vi "UI_playerWins.vi"(8 "error in (no error)":errorcluster, 11 "Array":refnum<vi>[](array[refnum])) -> (0 "error out":errorcluster, 3 "win string":string)   [LabVIEW 2020]
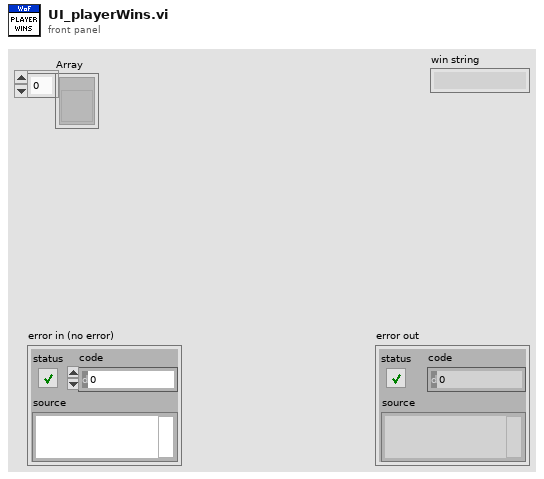
[diagram p1: front panel]
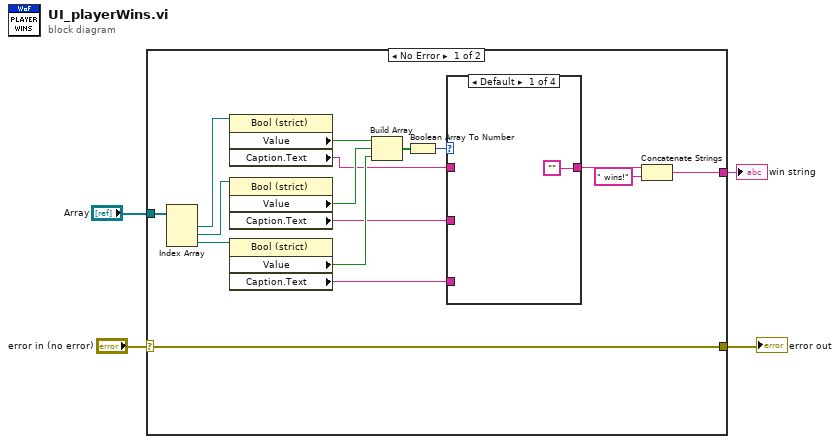
[diagram p0: block diagram]
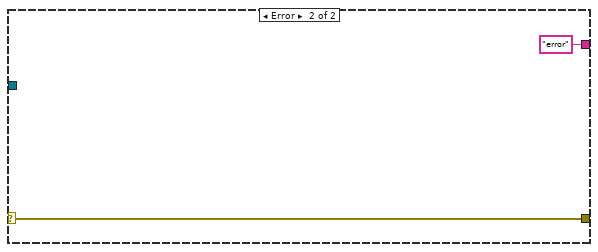
[diagram p5: hidden frame]
diagram:
  n1 = case shown="No Error" "error in (no error)" {
    selector: "error in (no error)" -> [w12 w26]
    tunnel: "Array" -> [w20 _]
    tunnel: [w12 w26] -> w2
    tunnel: [w5 "error"] -> w1
    frame No Error {
      n2 = Index Array(array=w20) -> (element #1=w19:refnum<vi>, element #2=w18:refnum<vi>, element #3=w17:refnum<vi>)  [unwired: 3 in]
      n3 = property class="Bool (strict)"(reference=w19) -> ("Value"=w16:bool, "Caption.Text"=w10:string)  [unwired: 1 in, 2 out]
      n4 = property class="Bool (strict)"(reference=w18) -> ("Value"=w15:bool, "Caption.Text"=w9:string)  [unwired: 1 in, 2 out]
      n5 = property class="Bool (strict)"(reference=w17) -> ("Value"=w14:bool, "Caption.Text"=w8:string)  [unwired: 1 in, 2 out]
      n6 = Build Array(w16, w15, w14) -> (w13:bool[])
      n7 = Boolean Array To Number(Boolean array=w13) -> (number=w11:u32)
      n8 = case shown="Default" w11 {
        tunnel: w10 -> [_ w22 _ _]
        tunnel: w9 -> [_ _ w23 _]
        tunnel: w8 -> [_ _ _ w24]
        tunnel: ["" w22 w23 w24] -> w7
        frame Default {
        }
        frame 1 {
        }
        frame 2 {
        }
        frame 4 {
        }
      }
      n9 = Concatenate Strings(w7, " wins!" ("string")) -> (w5:string)
    }
    frame Error {
    }
  }
  "error out" <- w2
  "win string" <- w1
